vi "Read Slicer Data.vi"() -> ()   [LabVIEW 2016]
uses:
  <vilib>/Utility/file.llb/Read Delimited Spreadsheet (DBL).vi
panel:
  out "Bead command":string
  out "All beads":dbl[][][](array[numeric])
  out "Raw slicer coordinates":string
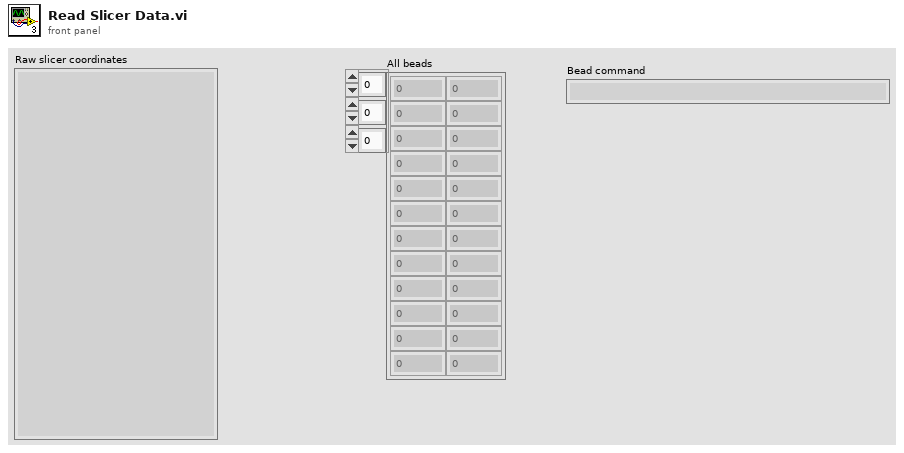
[diagram p1: front panel]
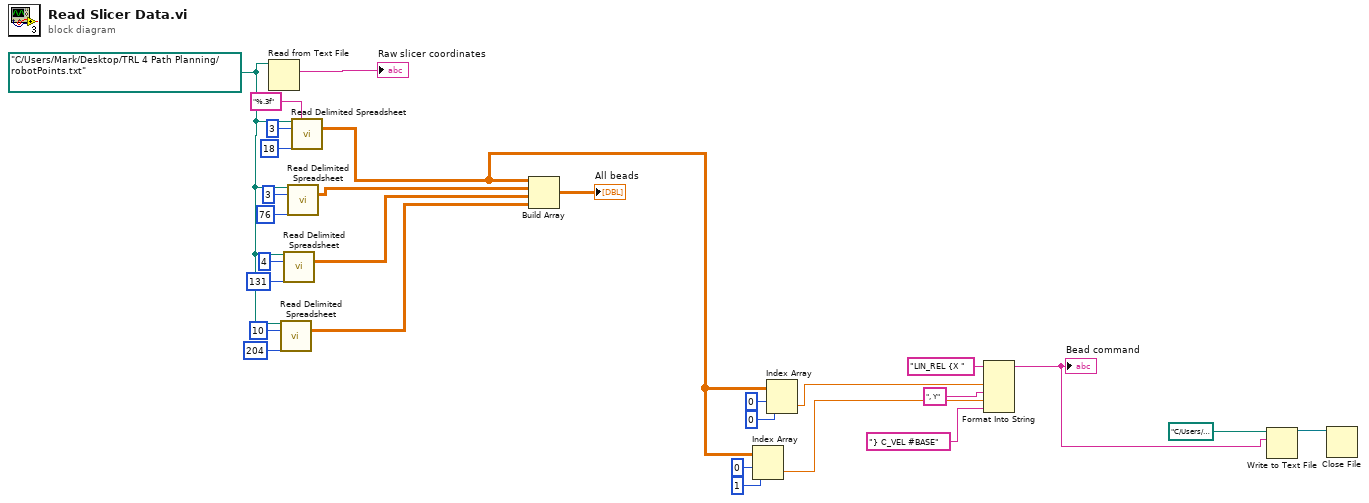
[diagram p0: block diagram]
diagram:
  w24 = path "C:/Users/Mark/Desktop/TRL 4 Path Planning/robotPoints.txt" ("file (use dialog)")
  n1 = Read from Text File(file (use dialog)=w24) -> (text=→"Raw slicer coordinates":string)  [unwired: 3 in, 3 out]
  n2 = call-poly <vilib>:"Read Delimited Spreadsheet.vi"("file path (dialog if empty)"=w24, "number of rows (all:-1)"=10, "start of read offset (chars.:0)"=204) -> ("all rows"=w15:dbl[][])  [unwired: 7 in, 5 out]
  n3 = call-poly <vilib>:"Read Delimited Spreadsheet.vi"("file path (dialog if empty)"=w24, "number of rows (all:-1)"=4, "start of read offset (chars.:0)"=131) -> ("all rows"=w16:dbl[][])  [unwired: 7 in, 5 out]
  n4 = call-poly <vilib>:"Read Delimited Spreadsheet.vi"("file path (dialog if empty)"=w24, "number of rows (all:-1)"=3, "start of read offset (chars.:0)"=76) -> ("all rows"=w17:dbl[][])  [unwired: 7 in, 5 out]
  n5 = call-poly <vilib>:"Read Delimited Spreadsheet.vi"("file path (dialog if empty)"=w24, "format (%.3f)"="%.3f", "number of rows (all:-1)"=3, "start of read offset (chars.:0)"=18) -> ("all rows"=w8:dbl[][])  [unwired: 6 in, 5 out]
  n6 = Build Array(w8, w17, w16, w15) -> (→"All beads":dbl[][][])
  n7 = Index Array(array=w8, index (row)=0, index (col)=1 ("disabled index (col)")) -> (element=w5:dbl)
  n8 = Index Array(array=w8, index (row)=0, index (col)=0 ("disabled index (col)")) -> (element=w10:dbl)
  n9 = Format Into String(initial string="LIN_REL {X ", w10, ", Y" ("initial string"), w5, "} C_VEL #BASE" ("initial string")) -> (resulting string=w2:string)  [unwired: 2 in, 1 out]
  "Bead command" <- w2
  n10 = Write to Text File(file (use dialog)=path "C:/Users/Mark/Desktop/TRL 4 Path Planning/TRL4Paths.txt", text=w2) -> (refnum out=w1:refnum<file>)  [unwired: 2 in, 2 out]
  n11 = Close File(refnum=w1) -> ()  [unwired: 1 in, 2 out]
